vi "GetValue.vi"(8 "error in":errorcluster, 11 "DateTime in":refnum<class "DateTime.lvclass">) -> (0 "error out":errorcluster, 2 "Value":timestamp, 3 "DateTime out":refnum<class "DateTime.lvclass">)   [LabVIEW 2021, in "ProligentXMLGenerator.lvlib" / "DateTime.lvclass"]
uses:
  DateTime.lvclass
  DateTime.lvclass/DateTime.ctl
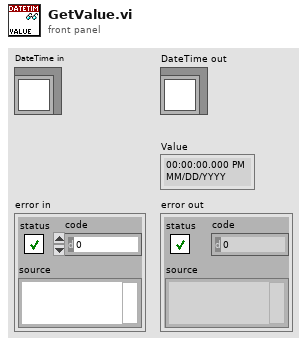
[diagram p1: front panel]
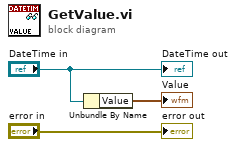
[diagram p0: block diagram]
diagram:
  n1 = Unbundle By Name("DateTime in") -> ("Value"=→"Value":timestamp)
  "error out" <- "error in"
  "DateTime out" <- "DateTime in"
